vi "条件结构.vi"() -> ()   [LabVIEW 2017]
panel:
  in  "字符串 3":string="你考试通过了"
  in  "字符串 2":string="输入错误"
  in  "字符串":string="你没有通过考试"
  out "温馨提示":string
  in  "请输入成绩":dbl
  in  "停止":bool
  out "恭喜":bool
  out "通过":bool
  out "输入错误":bool
  out "警告":bool
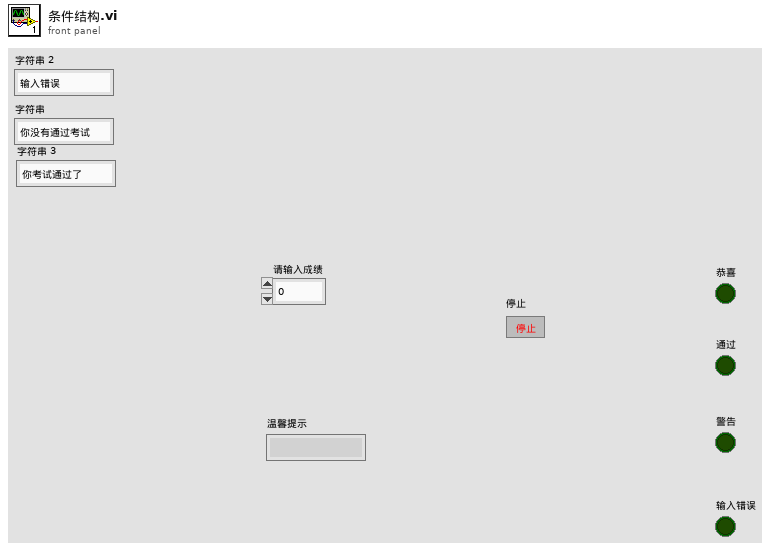
[diagram p1: front panel]
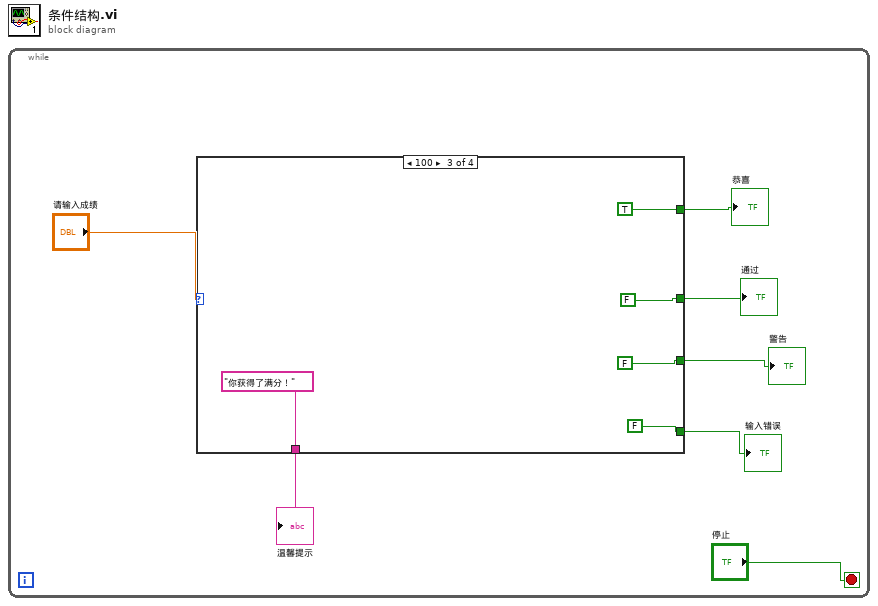
[diagram p0: block diagram]
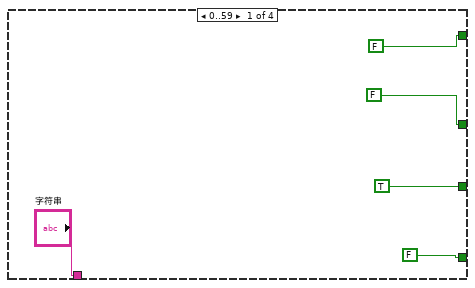
[diagram p2: hidden frame]
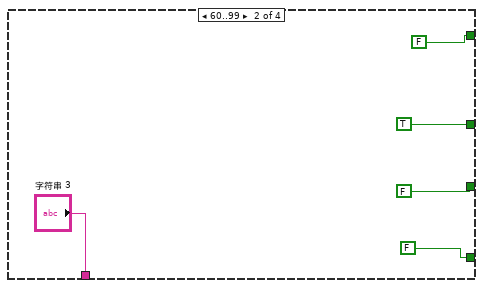
[diagram p3: hidden frame]
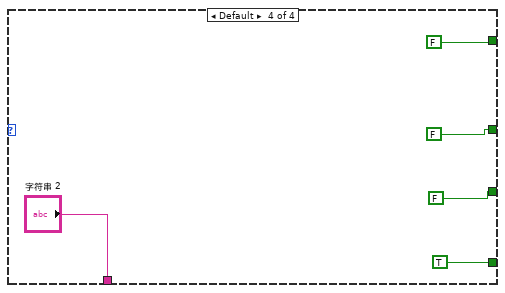
[diagram p4: hidden frame]
diagram:
  n1 = while {
    stop <- "停止" stop-if-true
    n2 = case shown="100" "请输入成绩" {
      tunnel: [FALSE FALSE FALSE TRUE] -> w6
      tunnel: ["字符串" "字符串 3" "你获得了满分！" "字符串 2"] -> w5
      tunnel: [TRUE FALSE FALSE FALSE] -> w4
      tunnel: [FALSE TRUE FALSE FALSE] -> w3
      tunnel: [FALSE FALSE TRUE FALSE] -> w2
      frame 0..59 {
      }
      frame 60..99 {
      }
      frame 100 {
      }
      frame Default {
      }
    }
    "警告" <- w4
    "输入错误" <- w6
    "通过" <- w3
    "恭喜" <- w2
    "温馨提示" <- w5
  }
